vi "_UploadFirmware.vi"() -> ()   [LabVIEW 2016]
panel:
  out "name":string
  in  "Connect REPL":bool
  in  "Test":bool
  in  "Stop":bool
  in  "Connect":bool
  in  "VISA Refnum in":refnum<visa-resource-name>="ASRL32::INSTR"
  in  "Stage 2":bool
  in  "Stage 1":bool
  in  "Copy":bool
  out "PC files":string[](array[string])=["fwupdate.mpy", "PYBD_SF2_W4F2.dfu.gz", "PYBD_SF2_W4F2_mboot.dfu.gz"]
  out "Console":string="\r\n>>> \r\nPYB: sync filesystems\r\nPYB: soft reboot\r\nMicroPython v1.10-210-g45076ee50-dirty on 2019-02-02; PYBD_SF2 with STM32F722IEK\r\nType \"help()\" for more information.\r\n>>> \r\n>>> import fwupdate\r\n>>> fwupdate.stage1()\r\nLoading file /flash/PYBD_SF2_W4F2_mboot.dfu.gz\r\nSupplied version of mboot is already on device.\r\nstage1 done, rebooting\r\nMicroPython v1.10-210-g45076ee50-dirty on 2019-02-02; PYBD_SF2 with STM32F722IEK\r\nType \"help()\" for more information.\r\n>>> \r\n>>> import fwupdate\r\n>>> fwupdate.stage2()\r\nstage2 done\r\n>>> \r\nPYB: sync filesystems\r\nPYB: soft reboot\r\nMicroPython v1.10-210-g45076ee50-dirty on 2019-02-02; PYBD_SF2 with STM32F722IEK\r\nType \"help()\" for more information.\r\n>>> \r\n>>> "
  # "1. Select your serial port\n2. connect up\n3. copy over the files to the Pyboard - and wait for them  \n          to copy over (it takes 30 sec)\n4. flash stage 1 - and wait for the lights to stop blinking (\n          it takes 30 sec)\n5. flash stage 2 and run a test"
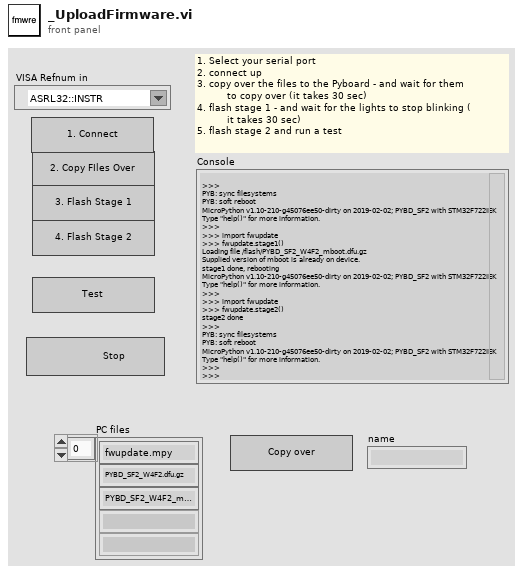
[diagram p1: front panel]
types:
  T1 = enum8{"Enabled", "Disabled", "Disabled and Grayed Out"}
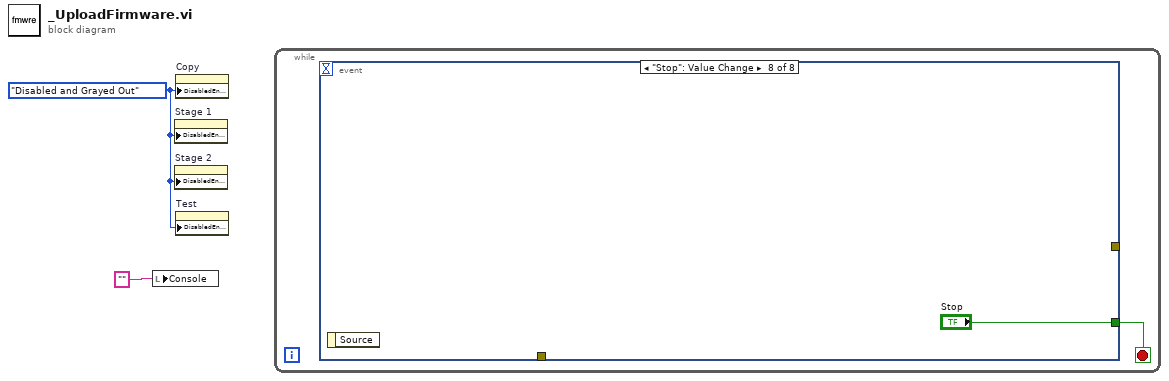
[diagram p0: block diagram]
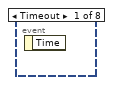
[diagram p2: hidden frame]
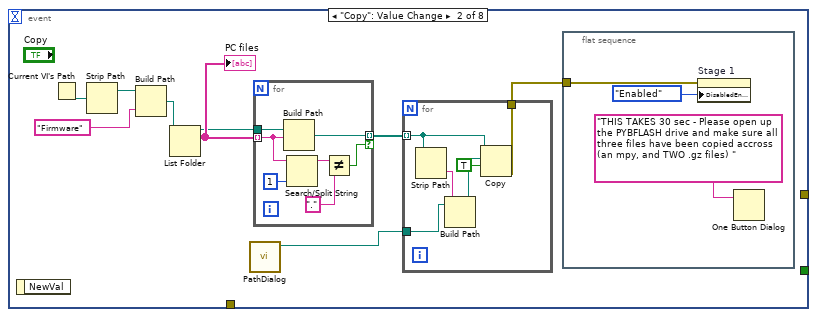
[diagram p3: hidden frame]
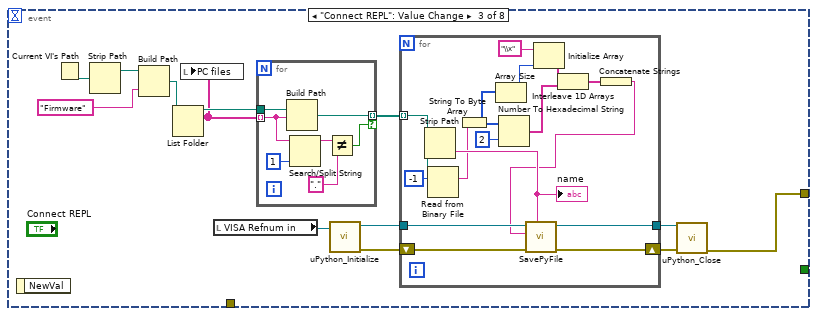
[diagram p4: hidden frame]
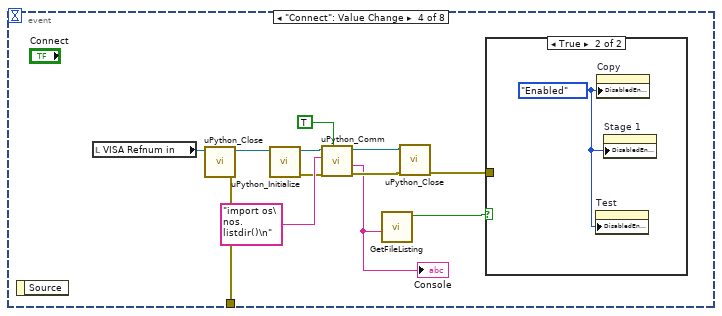
[diagram p5: hidden frame]
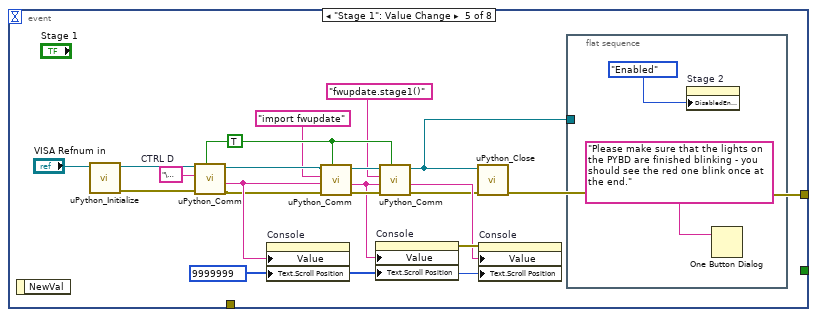
[diagram p7: hidden frame]
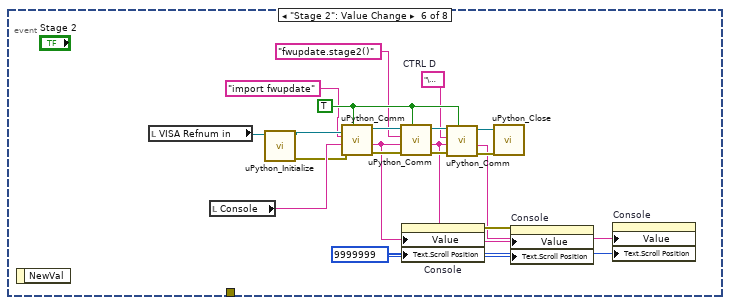
[diagram p8: hidden frame]
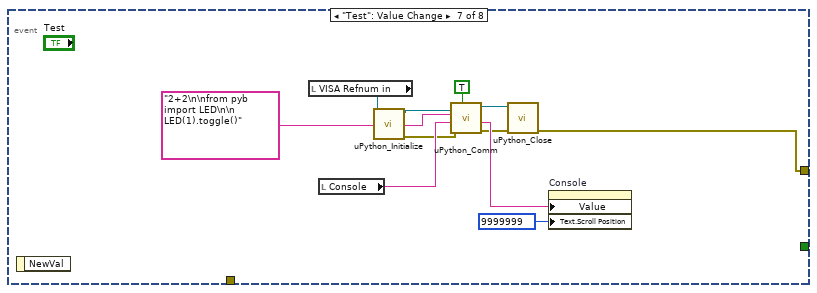
[diagram p9: hidden frame]
diagram:
  w2 = T1."Disabled and Grayed Out" ("Disabled")
  n1 = local write "Console"("") -> ()
  n2 = property on="Stage 1" class="Bool"("DisabledEnum"=w2) -> ()  [unwired: 2 in, 2 out]
  n3 = property on="Stage 2" class="Bool"("DisabledEnum"=w2) -> ()  [unwired: 2 in, 2 out]
  n4 = property on="Copy" class="Bool"("DisabledEnum"=w2) -> ()  [unwired: 2 in, 2 out]
  n5 = property on="Test" class="Bool"("DisabledEnum"=w2) -> ()  [unwired: 2 in, 2 out]
  n6 = while {
    stop <- w3 stop-if-true
    n7 = event shown="[7] \"Stop\": Value Change" {
      selector: _ -> [_ _ _ _ _ _ _ _]
      dyn-events: _ -> [_ _ _ _ _ _ _ _]
      timeout: _ -> [_ _ _ _ _ _ _ _]
      tunnel: [_ _ _ _ _ _ _ "Stop"] -> w3
      tunnel: [_ _ w29 _ w87 _ w118 _] -> _
      tunnel: [_ _ _ w66 _ _ _ _] -> _
      event Timeout {
        n8 = event-data() -> ()  [unwired: 1 in, 1 out]
      }
      event "Copy": Value Change {
        n9 = event-data() -> ()  [unwired: 1 in, 1 out]
        n10 = Current VI's Path() -> (path=w9:path)
        n11 = Strip Path(path=w9) -> (stripped path=w6:path)  [unwired: 1 out]
        n12 = Build Path(base path=w6, name or relative path="Firmware") -> (appended path=w5:path)
        n13 = List Folder(path=w5) -> (path out=w10:path, filenames=w11:string[])  [unwired: 3 in, 2 out]
        "PC files" <- w11
        n14 = call "PathDialog.vi"() -> ("Path 2out"=w4:path)  [unwired: 11 in]
        n15 = for {
          tunnel: w10 -> [w28]
          tunnel: w11 -> [w26] mode=indexing
          tunnel: [w27] -> w12 mode=indexing if=w22
          n16 = Build Path(base path=w28, name or relative path=w26) -> (appended path=w27:path)
          n17 = Search/Split String(string=w26, offset (0)=1) -> (substring before match=w24:string)  [unwired: 1 in, 2 out]
          n18 = Not Equal?(x=w24, y=".") -> (x != y?=w22:bool)
        }
        n19 = for {
          tunnel: w12 -> [w21] mode=indexing
          tunnel: w4 -> [w20]
          tunnel: [w16] -> w7
          n20 = Strip Path(path=w21) -> (name=w19:string)  [unwired: 1 out]
          n21 = Build Path(base path=w20, name or relative path=w19) -> (appended path=w18:path)
          n22 = Copy(9:TRUE ("overwrite (F)"), 10:w18, 11:w21) -> (0:w16:errorcluster)  [unwired: 2 in, 2 out]
        }
        n23 = flat-sequence {
          tunnel: w7 -> [w14]
          frame #0 {
            n24 = property on="Stage 1" class="Bool"(error in=w14, "DisabledEnum"=T1."Enabled" ("Disabled")) -> ()  [unwired: 1 in, 2 out]
            n25 = One Button Dialog(message="THIS TAKES 30 sec - Please open up the PYBFLASH drive and make sure all three files have been copied accross (an mpy, and TWO .gz files) ") -> ()  [unwired: 1 in, 1 out]
          }
        }
      }
      event "Connect REPL": Value Change {
        n26 = event-data() -> ()  [unwired: 1 in, 1 out]
        n27 = Current VI's Path() -> (path=w37:path)
        n28 = Strip Path(path=w37) -> (stripped path=w38:path)  [unwired: 1 out]
        n29 = Build Path(base path=w38, name or relative path="Firmware") -> (appended path=w40:path)
        n30 = List Folder(path=w40) -> (path out=w39:path, filenames=w35:string[])  [unwired: 3 in, 2 out]
        n31 = local write "PC files"(w35) -> ()
        n32 = local read "VISA Refnum in"() -> (w34:refnum<visa-resource-name>)
        n33 = for {
          tunnel: w39 -> [w64]
          tunnel: w35 -> [w62] mode=indexing
          tunnel: [w63] -> w41 mode=indexing if=w58
          n34 = Build Path(base path=w64, name or relative path=w62) -> (appended path=w63:path)
          n35 = Search/Split String(string=w62, offset (0)=1) -> (substring before match=w60:string)  [unwired: 1 in, 2 out]
          n36 = Not Equal?(x=w60, y=".") -> (x != y?=w58:bool)
        }
        n37 = call "uPython_Initialize.vi"("VISA Refnum in"=w34) -> ("error out"=w32:errorcluster, "VISA Refnum out"=w33:refnum<visa-resource-name>)  [unwired: 9 in]
        n38 = for {
          tunnel: w41 -> [w52] mode=indexing
          tunnel: w33 -> [w57]
          shift-right: [w55] -> w31
          shift-left: w32 -> [w56]
          tunnel: [w54] -> w30
          n39 = Strip Path(path=w52) -> (name=w53:string)  [unwired: 1 out]
          "name" <- w53
          n40 = Read from Binary File(10:-1 ("count (1)"), 11:w52) -> (2:w43:string)  [unwired: 4 in, 3 out]
          n41 = String To Byte Array(string=w43) -> (unsigned byte array=w47:u8[])
          n42 = Array Size(array=w47) -> (size(s)=w46:i32)
          n43 = Number To Hexadecimal String(1:i16 2 ("width (-)"), 2:w47) -> (0:w49:string[])
          n44 = Initialize Array("\\x" ("format string"), w46) -> (w45:string[])
          n45 = Interleave 1D Arrays(w45, w49) -> (w44:string[])
          n46 = Concatenate Strings(w44) -> (w42:string)
          n47 = call "SavePyFile.vi"("Name"=w53, "error in"=w56, "Python Code"=w42, "VISA in"=w57) -> ("error out"=w55:errorcluster, "VISA out"=w54:refnum<visa-resource-name>)  [unwired: 5 in, 1 out]
        }
        n48 = call "uPython_Close.vi"("error in"=w31, "VISA  in"=w30) -> ("error out"=w29:errorcluster)  [unwired: 8 in, 1 out]
      }
      event "Connect": Value Change {
        n49 = event-data() -> ()  [unwired: 1 in, 1 out]
        n50 = local read "VISA Refnum in"() -> (w75:refnum<visa-resource-name>)
        n51 = call "uPython_Close.vi"("VISA  in"=w75) -> ("error out"=w66:errorcluster, "VISA  out"=w76:refnum<visa-resource-name>)  [unwired: 9 in]
        n52 = call "uPython_Initialize.vi"("VISA Refnum in"=w76) -> ("error out"=w69:errorcluster, "VISA Refnum out"=w74:refnum<visa-resource-name>)  [unwired: 9 in]
        n53 = call "uPython_Comm.vi"("Wait for Reply?"=TRUE, "error in (no error)"=w69, "Script"="import os\nos.listdir()\n", "VISA Refnum in"=w74) -> ("error out"=w68:errorcluster, "Console Out"=w65:string, "VISA out"=w71:refnum<visa-resource-name>)  [unwired: 3 in, 2 out]
        "Console" <- w65
        n54 = call "GetFileListing.vi"("Console In"=w65) -> ("Success?"=w70:bool)  [unwired: 9 in, 1 out]
        n55 = call "uPython_Close.vi"("error in"=w68, "VISA  in"=w71) -> ("error out"=w67:errorcluster)  [unwired: 8 in, 1 out]
        n56 = case shown="True" w70 {
          tunnel: w67 -> [_ _]
          frame False {
          }
          frame True {
            w77 = T1."Enabled" ("Disabled")
            n57 = property on="Test" class="Bool"("DisabledEnum"=w77) -> ()  [unwired: 2 in, 2 out]
            n58 = property on="Copy" class="Bool"("DisabledEnum"=w77) -> ()  [unwired: 2 in, 2 out]
            n59 = property on="Stage 1" class="Bool"("DisabledEnum"=w77) -> ()  [unwired: 2 in, 2 out]
          }
        }
      }
      event "Stage 1": Value Change {
        w83 = u32 9999999 ("Text.Selection:End")
        w91 = TRUE ("Wait for Reply?")
        w88 = "\u0004"  # CTRL D
        n60 = event-data() -> ()  [unwired: 1 in, 1 out]
        n61 = call "uPython_Initialize.vi"("VISA Refnum in"="VISA Refnum in") -> ("error out"=w78:errorcluster, "VISA Refnum out"=w92:refnum<visa-resource-name>)  [unwired: 9 in]
        n62 = call "uPython_Comm.vi"("Wait for Reply?"=w91, "error in (no error)"=w78, "Script"=w88, "VISA Refnum in"=w92) -> ("error out"=w79:errorcluster, "Console Out"=w85:string, "VISA out"=w93:refnum<visa-resource-name>)  [unwired: 3 in, 2 out]
        n63 = property on="Console" class="Str"("Value"=w85, "Text.Scroll Position"=w83) -> ()  [unwired: 2 in, 2 out]
        n64 = call "uPython_Comm.vi"("Wait for Reply?"=w91, "error in (no error)"=w79, "Console In"=w85, "Script"="import fwupdate", "VISA Refnum in"=w93) -> ("error out"=w94:errorcluster, "Console Out"=w82:string, "VISA out"=w95:refnum<visa-resource-name>)  [unwired: 2 in, 2 out]
        n65 = property on="Console" class="Str"("Value"=w82, "Text.Scroll Position"=w83) -> (error out=w84:errorcluster)  [unwired: 2 in, 1 out]
        n66 = call "uPython_Comm.vi"("Wait for Reply?"=w91, "error in (no error)"=w94, "Console In"=w82, "Script"="fwupdate.stage1()", "VISA Refnum in"=w95) -> ("error out"=w80:errorcluster, "Console Out"=w81:string, "VISA out"=w86:refnum<visa-resource-name>)  [unwired: 2 in, 2 out]
        n67 = call "uPython_Close.vi"("error in"=w80, "VISA  in"=w86) -> ("error out"=w87:errorcluster)  [unwired: 8 in, 1 out]
        n68 = property on="Console" class="Str"(error in=w84, "Value"=w81, "Text.Scroll Position"=w83) -> ()  [unwired: 1 in, 2 out]
        n69 = flat-sequence {
          tunnel: w86 -> [_]
          frame #0 {
            n70 = property on="Stage 2" class="Bool"("DisabledEnum"=T1."Enabled" ("Disabled")) -> ()  [unwired: 2 in, 2 out]
            n71 = One Button Dialog(message="Please make sure that the lights on the PYBD are finished blinking - you should see the red one blink once at the end.") -> ()  [unwired: 1 in, 1 out]
          }
        }
      }
      event "Stage 2": Value Change {
        w100 = u32 9999999 ("Text.Selection:End")
        w111 = TRUE ("Wait for Reply?")
        w110 = "\u0004"  # CTRL D
        n72 = event-data() -> ()  [unwired: 1 in, 1 out]
        n73 = local read "VISA Refnum in"() -> (w105:refnum<visa-resource-name>)
        n74 = local read "Console"() -> (w107:string)
        n75 = call "uPython_Initialize.vi"("VISA Refnum in"=w105) -> ("error out"=w99:errorcluster, "VISA Refnum out"=w114:refnum<visa-resource-name>)  [unwired: 9 in]
        n76 = call "uPython_Comm.vi"("Wait for Reply?"=w111, "error in (no error)"=w99, "Console In"=w107, "Script"="import fwupdate", "VISA Refnum in"=w114) -> ("error out"=w113:errorcluster, "Console Out"=w102:string, "VISA out"=w112:refnum<visa-resource-name>)  [unwired: 2 in, 2 out]
        n77 = call "uPython_Comm.vi"("Wait for Reply?"=w111, "error in (no error)"=w113, "Console In"=w102, "Script"="fwupdate.stage2()", "VISA Refnum in"=w112) -> ("error out"=w106:errorcluster, "Console Out"=w103:string, "VISA out"=w115:refnum<visa-resource-name>)  [unwired: 2 in, 2 out]
        n78 = property on="Console" class="Str"("Value"=w102, "Text.Scroll Position"=w100) -> (error out=w104:errorcluster)  [unwired: 2 in, 1 out]
        n79 = call "uPython_Comm.vi"("Wait for Reply?"=w111, "error in (no error)"=w106, "Console In"=w103, "Script"=w110, "VISA Refnum in"=w115) -> ("error out"=w116:errorcluster, "Console Out"=w101:string, "VISA out"=w117:refnum<visa-resource-name>)  [unwired: 2 in, 2 out]
        n80 = call "uPython_Close.vi"("error in"=w116, "VISA  in"=w117) -> ()  [unwired: 8 in, 2 out]
        n81 = property on="Console" class="Str"(error in=w104, "Value"=w103, "Text.Scroll Position"=w100) -> ()  [unwired: 1 in, 2 out]
        n82 = property on="Console" class="Str"("Value"=w101, "Text.Scroll Position"=w100) -> ()  [unwired: 2 in, 2 out]
      }
      event "Test": Value Change {
        n83 = event-data() -> ()  [unwired: 1 in, 1 out]
        n84 = local read "VISA Refnum in"() -> (w125:refnum<visa-resource-name>)
        n85 = local read "Console"() -> (w126:string)
        n86 = call "uPython_Initialize.vi"("VISA Refnum in"=w125) -> ("error out"=w120:errorcluster, "VISA Refnum out"=w128:refnum<visa-resource-name>)  [unwired: 9 in]
        n87 = call "uPython_Comm.vi"("Wait for Reply?"=TRUE, "error in (no error)"=w120, "Console In"=w126, "Script"="2+2\n\nfrom pyb import LED\n\n     LED(1).toggle()", "VISA Refnum in"=w128) -> ("error out"=w119:errorcluster, "Console Out"=w121:string, "VISA out"=w123:refnum<visa-resource-name>)  [unwired: 2 in, 2 out]
        n88 = call "uPython_Close.vi"("error in"=w119, "VISA  in"=w123) -> ("error out"=w118:errorcluster)  [unwired: 8 in, 1 out]
        n89 = property on="Console" class="Str"("Value"=w121, "Text.Scroll Position"=u32 9999999 ("Text.Selection:End")) -> ()  [unwired: 2 in, 2 out]
      }
      event "Stop": Value Change {
        n90 = event-data() -> ()  [unwired: 1 in, 1 out]
      }
    }
  }
